vi "FPGA_DIOWriteSlowValueRelayRev.vi"(8 "error in (no error)":errorcluster, 10 "Relay Reverse":u8, 11 "DIODeviceRef In":T1) -> (0 "error out":errorcluster, 3 "DIODeviceRef Out":T1)   [LabVIEW 2017]
uses:
  <vilib>/Rock Robotics/SystemInterfaces/DIO/FPGA_DIODevRef.ctl
  <vilib>/Rock Robotics/SystemInterfaces/System/FPGA_SystemFPGA Ref Global.vi
  <vilib>/Utility/error.llb/Error Cluster From Error Code.vi
  <vilib>/rvi/errors/niLvFpgaAdjustHostInterfaceError.vi
  <vilib>/rvi/interface/nirviReadWriteControl/nirviReadWriteControl.xnode
  <vilib>/Rock Robotics/SystemInterfaces/System/FPGA_SystemFRC FPGA Ref.ctl
  <vilib>/rvi/interface/Simulation/niFpgaSimulationCallBeginRW.vi
  NiFpgaLv.dll
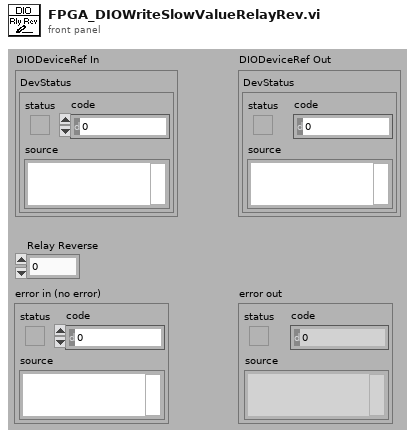
[diagram p1: front panel]
types:
  T1 = typedef "FPGA_DIODevRef.ctl" = cluster{"DevStatus":errorcluster}
  T2 = typedef "FPGA_SystemFRC FPGA Ref.ctl" = refnum<k20>
  T3 = cluster{"Forward":fxp<+,4,4>, "Reverse":fxp<+,4,4>}
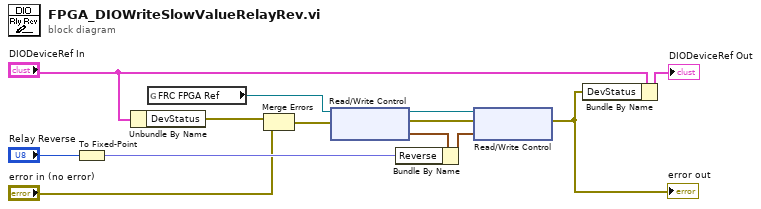
[diagram p0: block diagram]
diagram:
  n1 = To Fixed-Point(number="Relay Reverse") -> (fixed-point=w6:fxp<+,4,4>)  [unwired: 1 in]
  n2 = Unbundle By Name("DIODeviceRef In") -> ("DevStatus"=w8:errorcluster)
  n3 = global read "FPGA_SystemFPGA Ref Global.vi" "FRC FPGA Ref"() -> (w9:T2)
  n4 = Merge Errors(w8, "error in (no error)") -> (w7:errorcluster)
  n5 = xnode "Read/Write Control"("FPGA VI Reference In"=w9, "error in"=w7) -> ("FPGA VI Reference Out"=w5:T2, "error out"=w4:errorcluster, "Relay.Value"=w3:T3)
  n6 = Bundle By Name(cluster=w3, "Reverse"=w6) -> (w2:T3)
  n7 = xnode "Read/Write Control"("FPGA VI Reference In"=w5, "error in"=w4, "Relay.Value"=w2) -> ("error out"=w10:errorcluster)  [unwired: 1 out]
  "error out" <- w10
  n8 = Bundle By Name(cluster="DIODeviceRef In", "DevStatus"=w10) -> (→"DIODeviceRef Out":T1)
